vi "PH_Sixpack.Baud Converter.vi"(1 "BaudRate(19200)":u16=19200) -> (0 "BaudRate (19200)":enum32{"9600", "19200", "38400", "57600"}(ring))   [LabVIEW 2014, in "PH_Sixpack.lvlib"]
doc: "Converts the incoming Baud rate into the related ring entry; 19200 is default."
uses:
  PH_Sixpack.lvlib
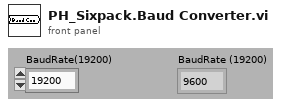
[diagram p1: front panel]
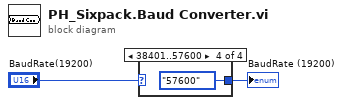
[diagram p0: block diagram]
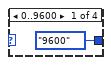
[diagram p2: hidden frame]
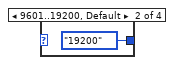
[diagram p3: hidden frame]
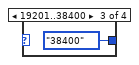
[diagram p4: hidden frame]
diagram:
  n1 = case shown="38401..57600" "BaudRate(19200)" {
    tunnel: [enum32{"9600", "19200", "38400", "57600"}."9600" ("BaudRate (19200)") enum32{"9600", "19200", "38400", "57600"}."19200" ("BaudRate (19200)") enum32{"9600", "19200", "38400", "57600"}."38400" ("BaudRate (19200)") enum32{"9600", "19200", "38400", "57600"}."57600" ("BaudRate (19200)")] -> w1
    frame 0..9600 {
    }
    frame 9601..19200, Default {
    }
    frame 19201..38400 {
    }
    frame 38401..57600 {
    }
  }
  "BaudRate (19200)" <- w1
